vi "Tetromino_MoveLeft.vi"(2 "Origin":i16) -> (16 "NewOrigin":i16)   [LabVIEW 2018]
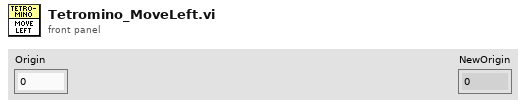
[diagram p1: front panel]
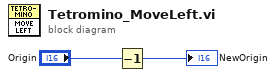
[diagram p0: block diagram]
diagram:
  n1 = Decrement(x="Origin") -> (x-1=→"NewOrigin":i16)
